vi "Diode-Load-Keywords.vi"() -> (2 "Diodes Keywords Array":T1[](array[typedef]))   [LabVIEW 2020]
uses:
  Diode-Keyword.ctl
  <vilib>/Utility/file.llb/Read Delimited Spreadsheet (string).vi
panel:
  out "Path to Keywords CSV":path
  out "Array":string[](array[string])
  out "subarray 2":string[][](array[string])
  out "subarray":string[](array[string])
  out "all rows":string[][](array[string])
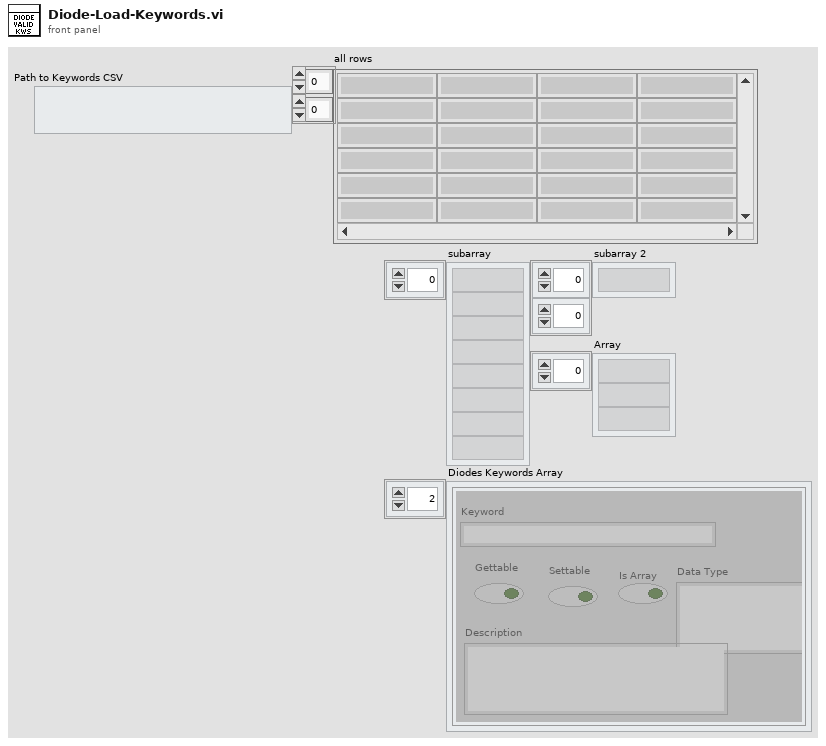
[diagram p1: front panel]
types:
  T1 = typedef "Diode-Keyword.ctl" = cluster{"Keyword":string, "Gettable":bool, "Settable":bool, "Is Array":bool, "Data Type":string, "Description":string}
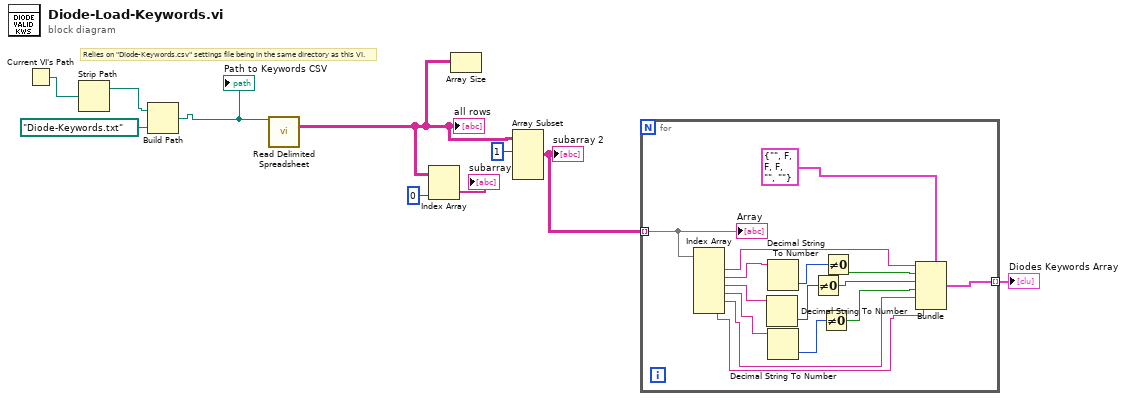
[diagram p0: block diagram]
diagram:
  # "Relies on \"Diode-Keywords.csv\" settings file being in the same directory as this VI."
  n1 = Current VI's Path() -> (path=w2:path)
  n2 = Strip Path(path=w2) -> (stripped path=w1:path)  [unwired: 1 out]
  n3 = Build Path(base path=w1, name or relative path=path "Diode-Keywords.txt") -> (appended path=w4:path)
  "Path to Keywords CSV" <- w4
  n4 = call-poly <vilib>:"Read Delimited Spreadsheet.vi"("file path (dialog if empty)"=w4) -> ("all rows"=w8:string[][])  [unwired: 9 in, 5 out]
  "all rows" <- w8
  n5 = Index Array(array=w8, index (col)=0 ("disabled index (col)")) -> (element=→"subarray":string[])  [unwired: 1 in]
  n6 = Array Size(array=w8) -> ()  [unwired: 1 out]
  n7 = Array Subset(array=w8, index (row)=1 ("index")) -> (w6:string[][])  [unwired: 3 in]
  "subarray 2" <- w6
  n8 = for {
    tunnel: w6 -> [w25] mode=indexing
    tunnel: [w18] -> w5 mode=indexing
    n9 = Index Array(array=w25) -> (element #1=w15:string, element #2=w14:string, element #3=w19:string, element #4=w13:string, element #5=w16:string, element #6=w17:string)  [unwired: 6 in]
    n10 = Decimal String To Number(string=w19) -> (number=w21:i32)  [unwired: 2 in, 1 out]
    n11 = Decimal String To Number(string=w14) -> (number=w23:i32)  [unwired: 2 in, 1 out]
    n12 = Decimal String To Number(string=w13) -> (number=w12:i32)  [unwired: 2 in, 1 out]
    n13 = Not Equal To 0?(x=w21) -> (x != 0?=w20:bool)
    n14 = Not Equal To 0?(x=w12) -> (x != 0?=w11:bool)
    n15 = Not Equal To 0?(x=w23) -> (x != 0?=w22:bool)
    n16 = Bundle(cluster=T1 {"Keyword"="", "Gettable"=FALSE, "Settable"=FALSE, "Is Array"=FALSE, "Data Type"="", "Description"=""} ("Diode Keyword"), "Keyword"=w15, "Gettable"=w22, "Settable"=w20, "Is Array"=w11, "Data Type"=w16, "Description"=w17) -> (w18:T1)
    "Array" <- w25
  }
  "Diodes Keywords Array" <- w5
